vi "Multiple Queues.vi"(6 "Method":T2, 8 "error in":errorcluster, 9 "Functions":T3, 10 "Quenes":T1) -> (0 "error out":errorcluster, 1 "# elements in queue":i32, 2 "queue out":refnum<queue>)   [LabVIEW 2020]
uses:
  Def/Queue_Function Def.ctl
  Def/Queue_Method Def.ctl
  Def/Queue_Def.ctl
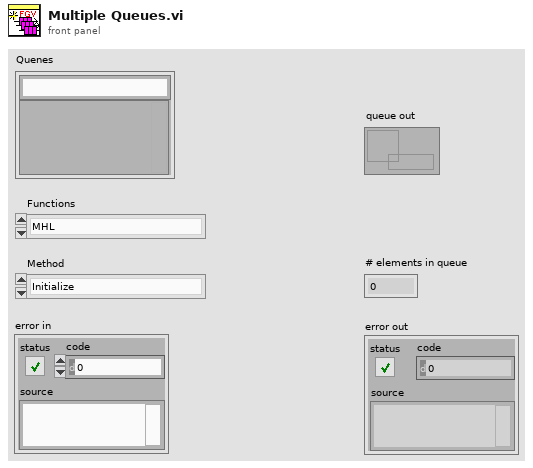
[diagram p1: front panel]
types:
  T1 = typedef "Queue_Def.ctl" = cluster{"Message":string, "Data":variant}
  T2 = typedef "Queue_Method Def.ctl" = enum16{"Initialize", "Read", "Write", "Insert", "Get_Specific_Quene_Status", "Flush Speciffic Quene", "Release All Quenes"}
  T3 = typedef "Queue_Function Def.ctl" = enum16{"MHL", "Return(Watch dog)", "Event Log", "Error Log"}
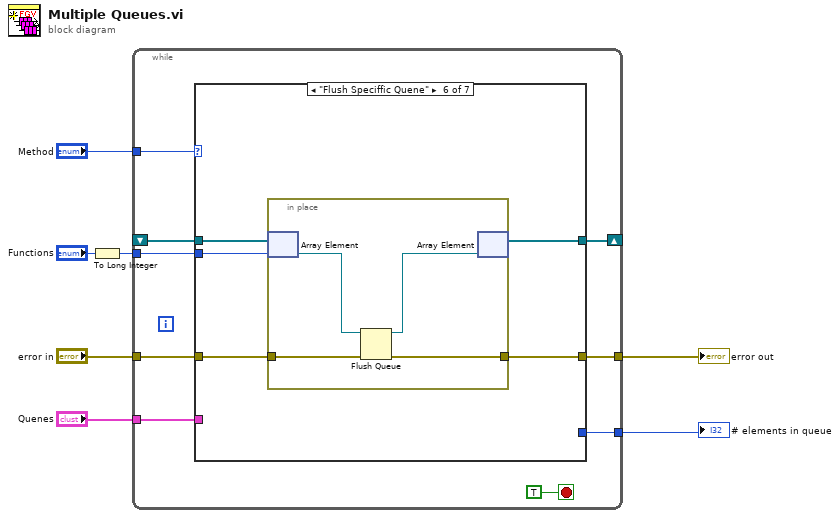
[diagram p0: block diagram]
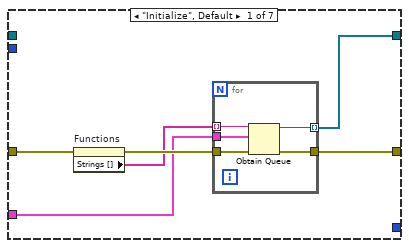
[diagram p2: hidden frame]
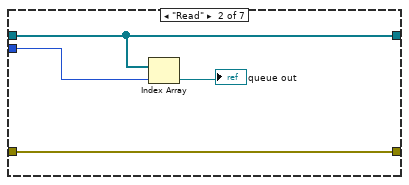
[diagram p3: hidden frame]
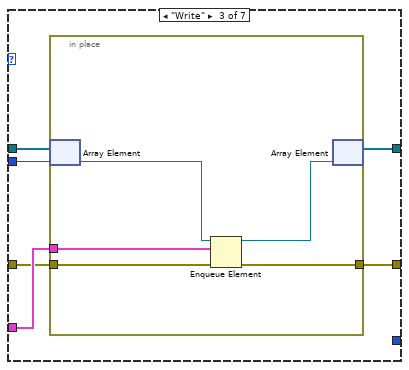
[diagram p4: hidden frame]
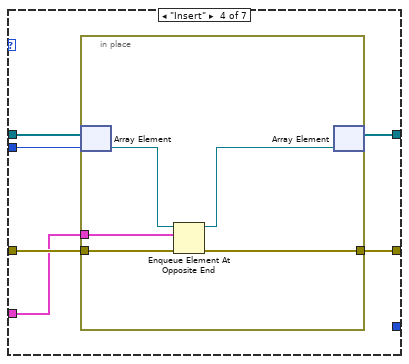
[diagram p5: hidden frame]
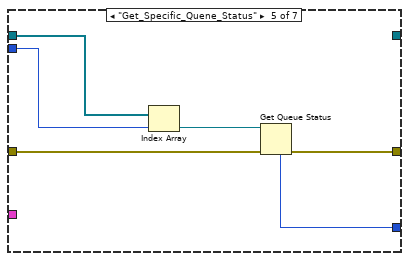
[diagram p6: hidden frame]
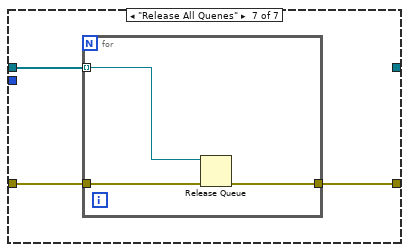
[diagram p7: hidden frame]
diagram:
  n1 = To Long Integer(number="Functions") -> (32bit integer=w2:i32)
  n2 = while {
    tunnel: "Method" -> [w15]
    tunnel: "error in" -> [w14]
    tunnel: [w13] -> w5
    shift-right: [w8] -> _
    shift-left: _ -> [w12]
    tunnel: "Quenes" -> [w11]
    tunnel: [w10] -> w3
    tunnel: w2 -> [w9]
    stop <- TRUE stop-if-true
    n3 = case shown="\"Flush Speciffic Quene\"" w15 {
      tunnel: w14 -> [w21 w31 w34 w47 w58 w63 w71]
      tunnel: [w22 w31 w33 w45 w57 w62 w70] -> w13
      tunnel: [w18 w28 w32 w43 _ w60 _] -> w8
      tunnel: w12 -> [_ w28 w37 w48 w55 w64 w69]
      tunnel: w11 -> [w17 _ w35 w46 _ _ _]
      tunnel: [_ _ _ _ w56 _ _] -> w10
      tunnel: w9 -> [_ w30 w36 w44 w54 w61 _]
      frame "Initialize", Default {
        n4 = property on="Functions" class="Enum (strict)"(error in=w21) -> (error out=w20:errorcluster, "Strings []"=w19:string[])  [unwired: 1 in, 1 out]
        n5 = for {
          tunnel: [w27] -> w22
          tunnel: [w26] -> w18 mode=indexing
          tunnel: w20 -> [w25]
          tunnel: w19 -> [w24] mode=indexing
          tunnel: w17 -> [w23]
          n6 = Obtain Queue(name (unnamed)=w24, element data type=w23, error in (no error)=w25) -> (queue out=w26:refnum<queue>, error out=w27:errorcluster)  [unwired: 2 in, 1 out]
        }
      }
      frame "Read" {
        n7 = Index Array(array=w28, index=w30) -> (element=→"queue out":refnum<queue>)
      }
      frame "Write" {
        n8 = in-place {
          in-place-border: w35 -> [w41]
          in-place-border: w34 -> [w40]
          in-place-border: [w39] -> w33
          n9 = in-place-array #1(w37, w36) -> (w42:refnum<queue>)
          n10 = Enqueue Element(queue=w42, element=w41, error in (no error)=w40) -> (queue out=w38:refnum<queue>, error out=w39:errorcluster)  [unwired: 1 in, 1 out]
          n11 = in-place-array #1(w38) -> (w32:refnum<queue>[])  [unwired: 1 out]
        }
      }
      frame "Insert" {
        n12 = in-place {
          in-place-border: [w52] -> w45
          in-place-border: w47 -> [w51]
          in-place-border: w46 -> [w53]
          n13 = in-place-array #2(w48, w44) -> (w50:refnum<queue>)
          n14 = Enqueue Element At Opposite End(queue=w50, element=w53, error in (no error)=w51) -> (queue out=w49:refnum<queue>, error out=w52:errorcluster)  [unwired: 1 in, 1 out]
          n15 = in-place-array #2(w49) -> (w43:refnum<queue>[])  [unwired: 1 out]
        }
      }
      frame "Get_Specific_Quene_Status" {
        n16 = Index Array(array=w55, index=w54) -> (element=w59:refnum<queue>)
        n17 = Get Queue Status(queue=w59, error in (no error)=w58) -> (error out=w57:errorcluster, # elements in queue=w56:i32)  [unwired: 1 in, 6 out]
      }
      frame "Flush Speciffic Quene" {
        n18 = in-place {
          in-place-border: w63 -> [w67]
          in-place-border: [w66] -> w62
          n19 = in-place-array #3(w64, w61) -> (w68:refnum<queue>)
          n20 = Flush Queue(queue=w68, error in (no error)=w67) -> (queue out=w65:refnum<queue>, error out=w66:errorcluster)  [unwired: 1 out]
          n21 = in-place-array #3(w65) -> (w60:refnum<queue>[])  [unwired: 1 out]
        }
      }
      frame "Release All Quenes" {
        n22 = for {
          tunnel: w71 -> [w74]
          tunnel: [w73] -> w70
          tunnel: w69 -> [w72] mode=indexing
          n23 = Release Queue(queue=w72, error in (no error)=w74) -> (error out=w73:errorcluster)  [unwired: 1 in, 2 out]
        }
      }
    }
  }
  "error out" <- w5
  "# elements in queue" <- w3
